vi "SBML_Sp_Param_Parser.vi"(8 "error in (no error)":errorcluster, 11 "Input SBML File":string) -> (0 "error out":errorcluster, 1 "Param Info":string[][](array[string]), 3 "Pr_Cnt":i32)   [LabVIEW 2014]
doc: "This VI extract the information of species' parameters present in SBML file. It takes the complete SBML file as input, and outputs: \nPr_Cnt --> How many parameters are there\nPr_Id_Arr --> Array of parameters\nPr_Name --> Array containing the name of parameters\nPr_Value --> Array containing the values of parameters\n\nDesigned by HB\nhaba@dtu.dk"
panel:
  out "Constant":string[](array[string])
  out "Units":string[](array[string])
  out "Pr_Value":string[](array[string])
  out "Pr_Name":string[](array[string])
  out "Pr_Id_Arr":string[](array[string])
  out "List of Parameters":string
  # "ID"
  # "Name"
  # "Value"
  # "Units"
  # "Constant"
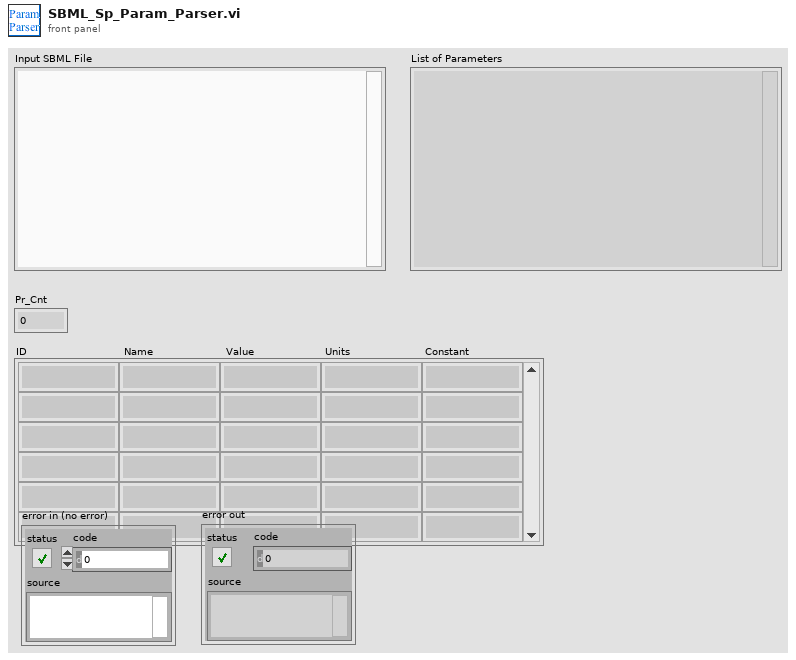
[diagram p1: front panel]
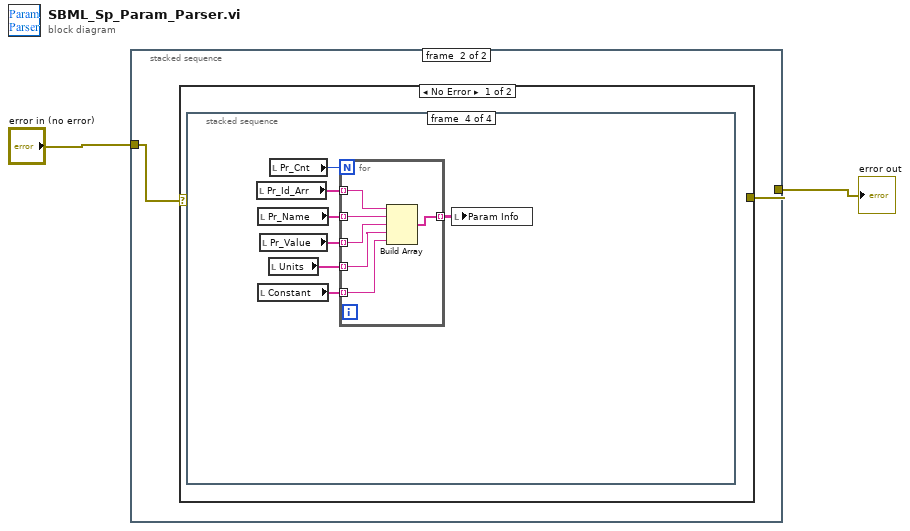
[diagram p0: block diagram]
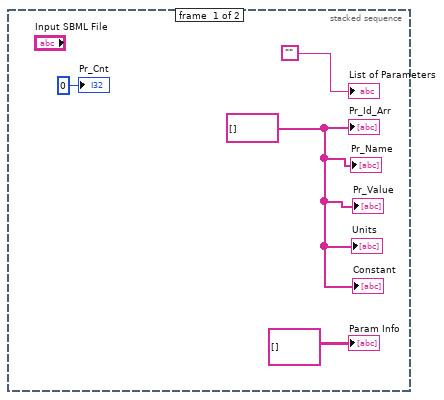
[diagram p2: hidden frame]
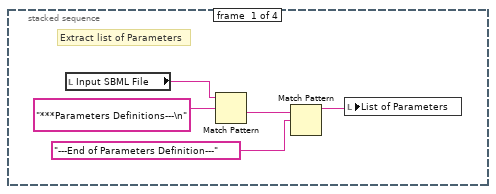
[diagram p3: hidden frame]
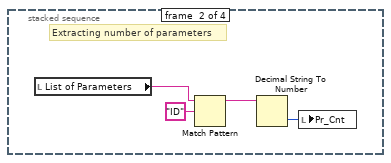
[diagram p4: hidden frame]
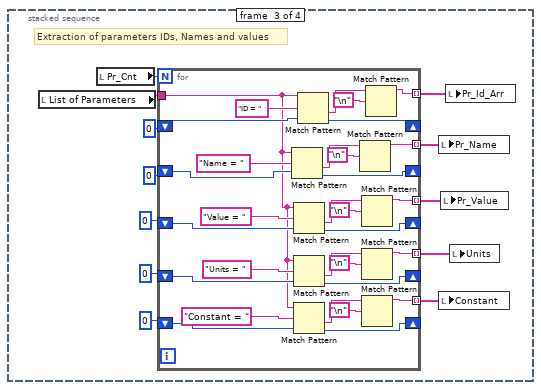
[diagram p5: hidden frame]
diagram:
  n1 = stacked-sequence {
    tunnel: "error in (no error)" -> [_ w7]
    tunnel: [_ w8] -> w1
    frame #0 {
      w3 = string[] [] ("Sp_Id_Arr")
      "List of Parameters" <- "" ("Full SBML File")
      "Pr_Cnt" <- 0 ("Sp_cnt")
      "Pr_Id_Arr" <- w3
      "Pr_Name" <- w3
      "Pr_Value" <- w3
      "Param Info" <- string[][] [] ("Param Info")
      "Units" <- w3
      "Constant" <- w3
    }
    frame #1 {
      n2 = case shown="No Error" w7 {
        selector: w7 -> [_ w74]
        tunnel: [_ w74] -> w8
        frame No Error {
          n3 = stacked-sequence {
            frame #0 {
              # "Extract list of Parameters"
              n4 = local read "Input SBML File"() -> (w12:string)
              n5 = Match Pattern(string=w12, regular expression="***Parameters Definitions---\n") -> (after substring=w10:string)  [unwired: 1 in, 3 out]
              n6 = Match Pattern(string=w10, regular expression="---End of Parameters Definition---") -> (before substring=w13:string)  [unwired: 1 in, 3 out]
              n7 = local write "List of Parameters"(w13) -> ()
            }
            frame #1 {
              # "Extracting number of parameters"
              n8 = local read "List of Parameters"() -> (w14:string)
              n9 = Match Pattern(string=w14, regular expression="ID") -> (before substring=w15:string)  [unwired: 1 in, 3 out]
              n10 = Decimal String To Number(string=w15) -> (number=w17:i32)  [unwired: 2 in, 1 out]
              n11 = local write "Pr_Cnt"(w17) -> ()
            }
            frame #2 {
              # "Extraction of parameters IDs, Names and values"
              n12 = local read "List of Parameters"() -> (w25:string)
              n13 = local read "Pr_Cnt"() -> (w24:i32)
              n14 = for {
                N: w24 -> [_]
                tunnel: w25 -> [w30]
                shift-right: [w56] -> _
                shift-left: 0 ("offset of match") -> [w55]
                tunnel: [w57] -> w27 mode=indexing
                shift-right: [w51] -> _
                shift-left: 0 ("offset past match") -> [w50]
                shift-right: [w46] -> _
                shift-left: 0 ("offset past match") -> [w45]
                tunnel: [w44] -> w23 mode=indexing
                tunnel: [w43] -> w22 mode=indexing
                shift-right: [w40] -> _
                shift-left: 0 ("offset past match") -> [w41]
                tunnel: [w42] -> w21 mode=indexing
                shift-right: [w33] -> _
                shift-left: 0 ("offset past match") -> [w32]
                tunnel: [w31] -> w18 mode=indexing
                n15 = Match Pattern(string=w30, regular expression="Name = ", offset (0)=w45) -> (after substring=w47:string, offset past match=w46:i32)  [unwired: 2 out]
                n16 = Match Pattern(string=w30, regular expression="Value = ", offset (0)=w50) -> (after substring=w54:string, offset past match=w51:i32)  [unwired: 2 out]
                n17 = Match Pattern(string=w30, regular expression="Units = ", offset (0)=w41) -> (after substring=w37:string, offset past match=w40:i32)  [unwired: 2 out]
                n18 = Match Pattern(string=w30, regular expression="Constant = ", offset (0)=w32) -> (after substring=w36:string, offset past match=w33:i32)  [unwired: 2 out]
                n19 = Match Pattern(string=w30, regular expression="ID = ", offset (0)=w55) -> (after substring=w58:string, offset past match=w56:i32)  [unwired: 2 out]
                n20 = Match Pattern(string=w47, regular expression="\n") -> (before substring=w43:string)  [unwired: 1 in, 3 out]
                n21 = Match Pattern(string=w54, regular expression="\n") -> (before substring=w44:string)  [unwired: 1 in, 3 out]
                n22 = Match Pattern(string=w37, regular expression="\n") -> (before substring=w42:string)  [unwired: 1 in, 3 out]
                n23 = Match Pattern(string=w36, regular expression="\n") -> (before substring=w31:string)  [unwired: 1 in, 3 out]
                n24 = Match Pattern(string=w58, regular expression="\n") -> (before substring=w57:string)  [unwired: 1 in, 3 out]
              }
              n25 = local write "Pr_Name"(w22) -> ()
              n26 = local write "Constant"(w18) -> ()
              n27 = local write "Pr_Value"(w23) -> ()
              n28 = local write "Pr_Id_Arr"(w27) -> ()
              n29 = local write "Units"(w21) -> ()
            }
            frame #3 {
              n30 = local read "Pr_Id_Arr"() -> (w63:string[])
              n31 = local read "Pr_Name"() -> (w65:string[])
              n32 = local read "Constant"() -> (w61:string[])
              n33 = local read "Pr_Value"() -> (w64:string[])
              n34 = local read "Units"() -> (w62:string[])
              n35 = local read "Pr_Cnt"() -> (w66:i32)
              n36 = for {
                N: w66 -> [_]
                tunnel: w63 -> [w73] mode=indexing
                tunnel: w65 -> [w72] mode=indexing
                tunnel: w64 -> [w71] mode=indexing
                tunnel: [w70] -> w67 mode=indexing
                tunnel: w62 -> [w69] mode=indexing
                tunnel: w61 -> [w68] mode=indexing
                n37 = Build Array(w73, w72, w71, w69, w68) -> (w70:string[])
              }
              n38 = local write "Param Info"(w67) -> ()
            }
          }
        }
        frame Error {
        }
      }
    }
  }
  "error out" <- w1
